vi "ACal-Create ER10B PTCal.vi"(5 "Mic Sens (dB V/SPL)":dbl) -> (15 "error out":errorcluster)   [LabVIEW 2020]
uses:
  Type Defs/Cal Stimulus.ctl
  Utility VIs/Math VIs/LinSpace (start-stop-step).vi
panel:
  in  "Resol":dbl=50.0 format="%#_13g"
  in  "Fs":dbl=100000.0 format="%#_13g"
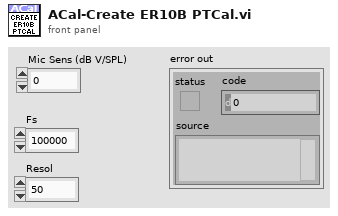
[diagram p1: front panel]
types:
  T1 = typedef "Cal Stimulus.ctl" = cluster{"Min Freq (Hz)":dbl, "Max Freq (Hz)":dbl, "Freq Step (Hz)":dbl, "Waveform":enum16{"Chirp", "Weighted"}, "Attenuation (dB)":dbl, "Sample Rate (Hz)":dbl}
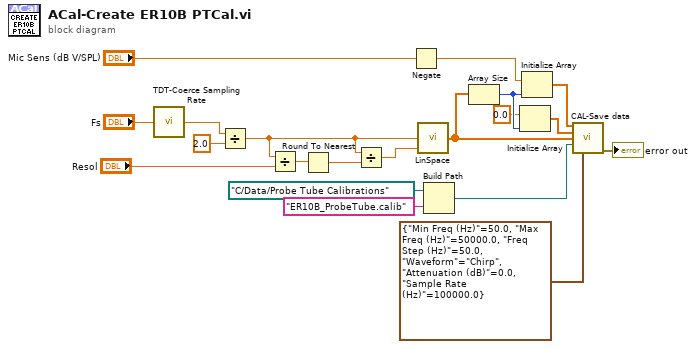
[diagram p0: block diagram]
diagram:
  n1 = call "TDT-Coerce Sampling Rate.vi"("Fs (Hz)"="Fs") -> ("Coerced"=w18:dbl)
  n2 = Divide(x=w18, y=2.0) -> (x/y=w13:dbl)
  n3 = Divide(x=w13, y="Resol") -> (x/y=w16:dbl)
  n4 = Round To Nearest(number=w16) -> (nearest integer value=w15:dbl)
  n5 = Divide(x=w13, y=w15) -> (x/y=w14:dbl)
  n6 = Negate(x="Mic Sens (dB V/SPL)") -> (-x=w1:dbl)
  n7 = call-poly "LinSpace.vi"("Step"=w14, "Stop"=w13) -> ("Array"=w12:dbl[])  [unwired: 2 in, 1 out]
  n8 = Build Path(base path=path "C:/Data/Probe Tube Calibrations", name or relative path="ER10B_ProbeTube.calib") -> (appended path=w3:path)
  n9 = Array Size(array=w12) -> (size(s)=w9:i32)
  n10 = Initialize Array(0.0 ("element"), w9) -> (w7:dbl[])
  n11 = Initialize Array(w1, w9) -> (w10:dbl[])
  n12 = call "CAL-Save data.vi"("Mag"=w10, "Phase"=w7, "Frequency"=w12, "path"=w3, "Cal Stimulus"=T1 {"Min Freq (Hz)"=50.0, "Max Freq (Hz)"=50000.0, "Freq Step (Hz)"=50.0, "Waveform"=enum."Chirp", "Attenuation (dB)"=0.0, "Sample Rate (Hz)"=100000.0}) -> ("error out"=→"error out":errorcluster)  [unwired: 9 in, 1 out]
